vi "Load Sequence Names.vi"(8 "error in (no error)":errorcluster, 10 "SequenceFile":refnum<class "SequenceFile.lvclass">, 11 "SequenceViewPanel in":refnum<class "SequenceViewPanel.lvclass">) -> (0 "error out":errorcluster, 3 "SequenceViewPanel out":refnum<class "SequenceViewPanel.lvclass">)   [LabVIEW 2020, in "TSnax UI.lvlib" / "SequenceViewPanel.lvclass"]
uses:
  SequenceViewPanel.lvclass
  TSnax/SequenceFile/SequenceFile.lvclass
  SequenceViewPanel.lvclass/SequenceViewPanel.ctl
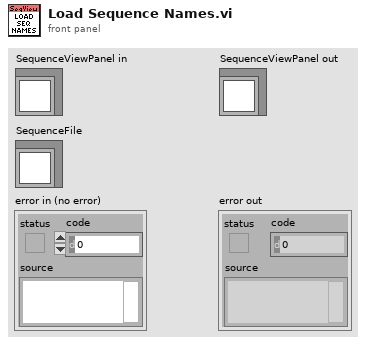
[diagram p1: front panel]
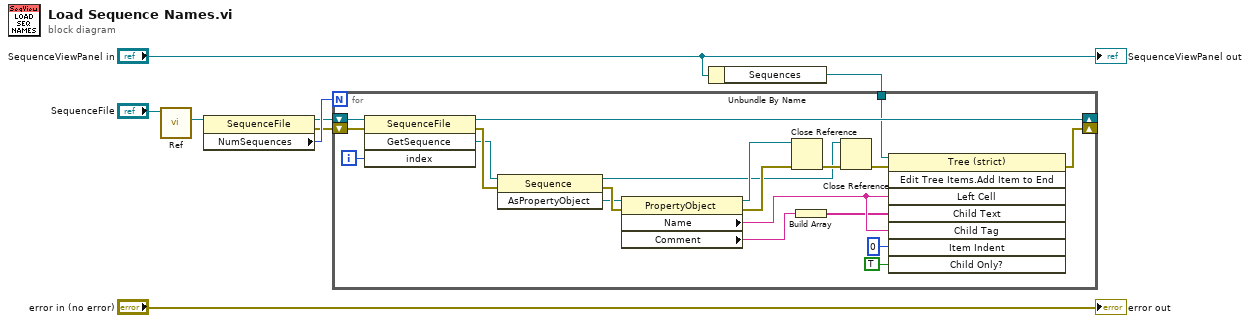
[diagram p0: block diagram]
diagram:
  n1 = call "Ref.vi"("SequenceFile in"="SequenceFile") -> ("Ref"=w7:refnum<k7>)  [unwired: 8 in, 2 out]
  n2 = property class="SequenceFile"(reference=w7) -> (reference out=w4:refnum<k7>, error out=w3:errorcluster, "NumSequences"=w5:i32)  [unwired: 1 in]
  n3 = Unbundle By Name("SequenceViewPanel in") -> ("Sequences"=w1:refnum<vi>)
  n4 = for {
    N: w5 -> [_]
    shift-right: [w23] -> _
    shift-left: w4 -> [w25]
    shift-right: [w17] -> _
    shift-left: w3 -> [w22]
    tunnel: w1 -> [w21]
    i -> [w24]
    n5 = invoke class="SequenceFile" method="GetSequence"(reference=w25, error in=w22, "index"=w24) -> (reference out=w23:refnum<k7>, error out=w26:errorcluster, "GetSequence"=w16:refnum<k7>)  [unwired: 1 in, 1 out]
    n6 = invoke class="Sequence" method="AsPropertyObject"(reference=w16, error in=w26) -> (reference out=w12:refnum<k7>, error out=w27:errorcluster, "AsPropertyObject"=w15:refnum<k7>)  [unwired: 1 in]
    n7 = property class="PropertyObject"(reference=w15, error in=w27) -> (reference out=w14:refnum<k7>, error out=w13:errorcluster, "Name"=w11:string, "Comment"=w10:string)
    n8 = Close Reference(reference=w14, error in (no error)=w13) -> (error out=w28:errorcluster)
    n9 = Build Array(w10) -> (w9:string[])
    n10 = Close Reference(reference=w12, error in (no error)=w28) -> (error out=w20:errorcluster)
    n11 = invoke class="Tree (strict)" method="Edit Tree Items.Add Item to End"(reference=w21, error in=w20, "Left Cell"=w11, "Child Text"=w9, "Child Tag"=w11, "Item Indent"=0 ("New Item Indentation"), "Child Only?"=TRUE) -> (error out=w17:errorcluster)  [unwired: 1 in, 7 out]
  }
  "error out" <- "error in (no error)"
  "SequenceViewPanel out" <- "SequenceViewPanel in"
